vi "Print Report ext.vi"(4 "IE Print Options":i32(ring)=1 items=["OLECMDEXECOPT_DODEFAULT", "OLECMDEXECOPT_PROMPTUSER", "OLECMDEXECOPT_DONTPROMPTUSER", "OLECMDEXECOPT_SHOWHELP"], 5 "error in (no error)":errorcluster, 6 "number of copies (1)":i32=1, 7 "printer name (default)":string, 8 "report in":T1) -> (1 "error out":errorcluster, 3 "report out":T1)   [LabVIEW 2017]
doc: "Prints a standard or HTML report to a designated printer or to the default printer on the computer.\n\nextended to allow option of opening IE print dialog for HTML reports"
uses:
  <vilib>/Utility/NIReport.llb/NI_ReportGenerationCore.lvlib
  <vilib>/Utility/NIReport.llb/NI_report.lvclass
  <vilib>/Utility/NIReport.llb/Generate Report Object Reference.ctl
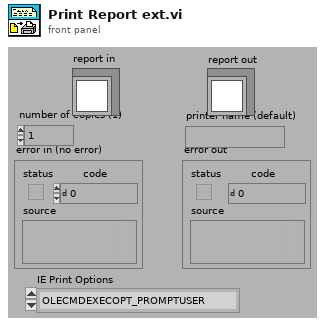
[diagram p1: front panel]
types:
  T1 = typedef "Generate Report Object Reference.ctl" = refnum<class "NI_report.lvclass">
  T2 = enum16{"Standard Report", "HTML", "Word", "Excel"}
  T3 = typedef "Generate Report Data Members.ctl" = cluster{"Title Text":string, "Header Text":string, "Body Text":string, "Footer Text":string, "Image List":string[], "NIReports.Report":refnum<k7>, "Report Type":enum16{"Standard Report", "HTML"}, "Font Tag":string}
  T4 = typedef "Generate Report Object Reference.ctl" = refnum<k1>
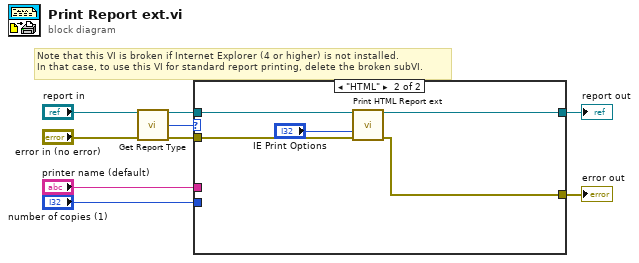
[diagram p0: block diagram]
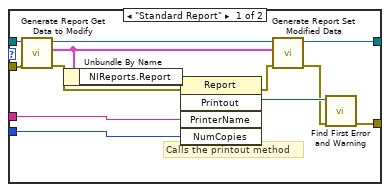
[diagram p2: hidden frame]
diagram:
  # "Note that this VI is broken if Internet Explorer (4 or higher) is not installed. \nIn that case, to use this VI for standard report printing, delete the broken subVI."
  n1 = call-dynamic "Get Report Type.vi"("report in"="report in", "error in (no error)"="error in (no error)") -> ("report out"=w3:T1, "report type"=w1:T2, "error out"=w2:errorcluster)  [unwired: 11 in]
  n2 = case shown="\"HTML\"" w1 {
    tunnel: "printer name (default)" -> [w22 _]
    tunnel: "number of copies (1)" -> [w21 _]
    tunnel: w3 -> [w20 w27]
    tunnel: w2 -> [w19 w26]
    tunnel: [w11 w25] -> w7
    tunnel: [w10 w24] -> w6
    frame "Standard Report" {
      # "Calls the printout method"
      n3 = call <vilib>:"Generate Report Get Data to Modify.vi"("error in (no error)"=w19, "report in"=w20) -> ("error out"=w17:errorcluster, "data"=w14:T3, "report out"=w15:T4)  [unwired: 2 in, 1 out]
      n4 = Unbundle By Name(w14) -> ("NIReports.Report"=w18:refnum<k7>)
      n5 = invoke class="Report" method="Printout"(reference=w18, error in=w17, "PrinterName"=w22, "NumCopies"=w21) -> (error out=w16:errorcluster, "Printout"=w13:i32)  [unwired: 1 in, 3 out]
      n6 = call <vilib>:"Generate Report Set Modified Data.vi"("error in (no error)"=w16, "data"=w14, "report in"=w15) -> ("error out"=w12:errorcluster, "report out"=w10:T4)  [unwired: 3 in]
      n7 = call <vilib>:"Find First Error and Warning.vi"("error in (no error)"=w12, "error code"=w13) -> ("error out"=w11:errorcluster)  [unwired: 4 in, 1 out]
    }
    frame "HTML" {
      n8 = call "Print HTML Report ext.vi"("report in"=w27, "IE Print Options"="IE Print Options", "error in (no error)"=w26) -> ("report out"=w24:T1, "error out"=w25:errorcluster)  [unwired: 11 in]
    }
  }
  "error out" <- w7
  "report out" <- w6
